vi "convert_doubleArray_to_string.vi"(2 "Max Elements Count (All)":i32=-1, 3 "Format string (%.;%#.12g)":string="%.;%#.12g", 4 "double array in":dbl[](array[numeric]) format="%#.12g", 5 "String to add before (\"\")":string) -> (1 "string out":string)   [LabVIEW 2014, in "rszvl_rsidr_core.lvlib"]
uses:
  rszvl_rsidr_core.lvlib
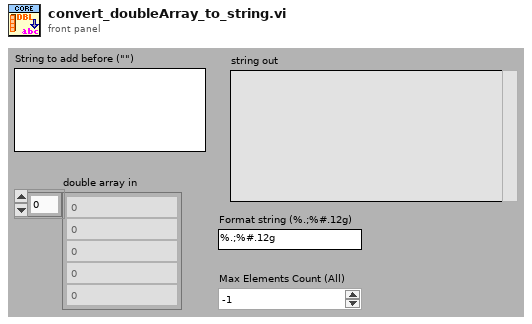
[diagram p1: front panel]
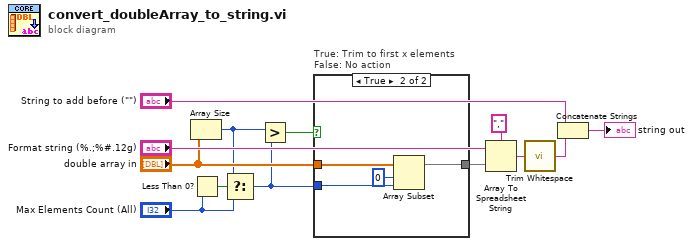
[diagram p0: block diagram]
diagram:
  n1 = Array Size(array="double array in") -> (size(s)=w4:i32)
  n2 = Less Than 0?(x="Max Elements Count (All)") -> (x < 0?=w6:bool)
  n3 = Select(t=w4, s=w6, f="Max Elements Count (All)") -> (s? t:f=w2:i32)
  n4 = Greater?(x=w4, y=w2) -> (0:w3:bool)
  n5 = case "True: Trim to first x elements\nFalse: No action" shown="True" w3 {
    tunnel: [w14 w15] -> w8
    tunnel: "double array in" -> [w14 w18]
    tunnel: w2 -> [_ w16]
    frame False {
    }
    frame True {
      n6 = Array Subset(array=w18, index=0, length=w16) -> (w15:dbl[])
    }
  }
  n7 = Array To Spreadsheet String(delimiter (Tab)=",", array=w8, 3:"Format string (%.;%#.12g)") -> (spreadsheet string=w11:string)
  n8 = call "Trim Whitespace.vi"("string"=w11) -> ("trimmed string"=w9:string)  [unwired: 1 in]
  n9 = Concatenate Strings("String to add before (\"\")", w9) -> (→"string out":string)
